vi "Initialize.vi"(8 "error in (no error)":errorcluster, 9 "Type":T1) -> (0 "error out":errorcluster, 1 "Stop Event":refnum<user-event>, 3 "UI_ProgressBar out":refnum<class "UI_ProgressDlg.lvclass">)   [LabVIEW 2014, in "UI_ProgressDlg.lvlib" / "UI_ProgressDlg.lvclass"]
uses:
  UI_ProgressDlg.lvclass
  _Control/DEF-Type.ctl
  _Control/DEF-Data.ctl
  UI_ProgressDlg.lvclass/UI_ProgressDlg.ctl
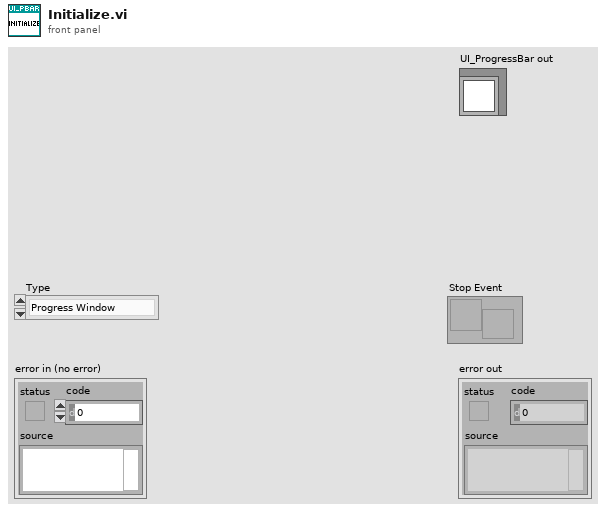
[diagram p1: front panel]
types:
  T1 = typedef "UI_ProgressDlg.lvlib/UI_ProgressDlg.lvclass/DEF-Type.ctl" = enum16{"Progress Window", "Buzy Window", "Timer Window"}
  T2 = typedef "UI_ProgressDlg.lvlib/UI_ProgressDlg.lvclass/DEF-Data.ctl" = cluster{"stopped?":bool}
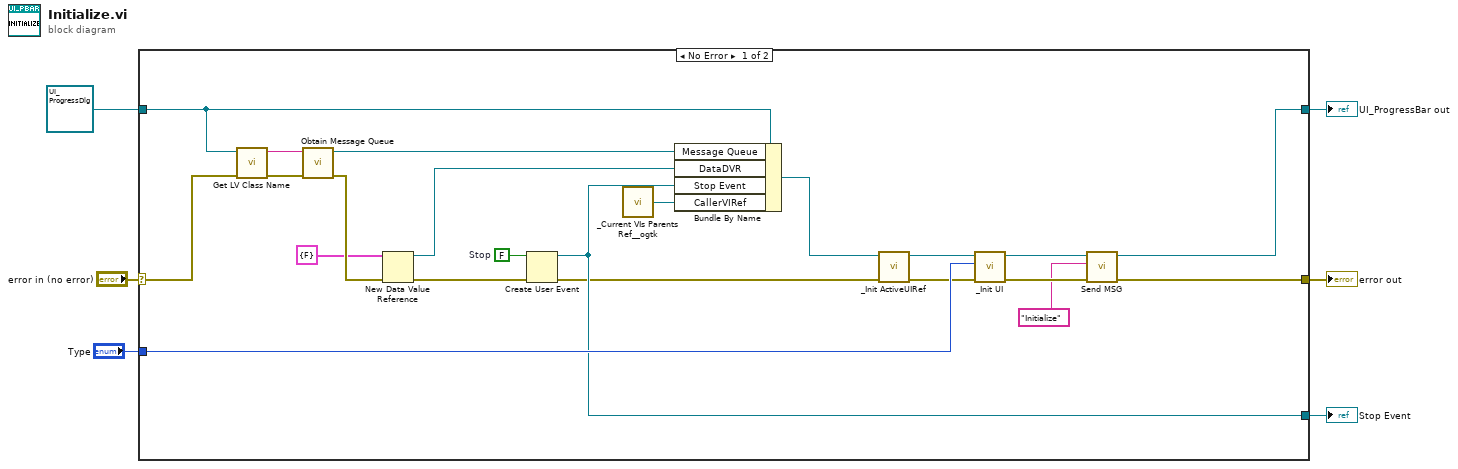
[diagram p0: block diagram]
diagram:
  n1 = case shown="No Error" "error in (no error)" {
    selector: "error in (no error)" -> [w28 w30]
    tunnel: [w17 w30] -> w5
    tunnel: [w19 w29] -> w3
    tunnel: refnum<class "UI_ProgressDlg.lvclass"> refnum ("UI_ProgressBar in") -> [w27 w29]
    tunnel: "Type" -> [w22 _]
    tunnel: [w13 _] -> w1
    frame No Error {
      w15 = FALSE  # Stop
      n2 = call <vilib>:"Get LV Class Name.vi"("error in (no error)"=w28, "object"=w27) -> ("error out"=w25:errorcluster, "class name"=w26:string)  [unwired: 8 in]
      n3 = call "Obtain Message Queue.vi"("error in (no error)"=w25, "name (unnamed)"=w26) -> ("error out"=w24:errorcluster, "Message Queue"=w23:refnum<queue>)  [unwired: 8 in]
      n4 = New Data Value Reference(data value=T2 {"stopped?"=FALSE} ("data"), error in=w24) -> (data value reference=w20:refnum<data-value>, error out=w14:errorcluster)
      n5 = Create User Event(user event datatype=w15, error in=w14) -> (user event=w13:refnum<user-event>, error out=w8:errorcluster)
      n6 = call "_Current VIs Parents Ref__ogtk.vi"() -> ("Calling VI's Reference"=w11:refnum<vi>)  [unwired: 2 in]
      n7 = Bundle By Name(cluster=w27, "Message Queue"=w23, "DataDVR"=w20, "Stop Event"=w13, "CallerVIRef"=w11) -> (w10:refnum<class "UI_ProgressDlg.lvclass">)
      n8 = call "_Init ActiveUIRef.vi"("error in (no error)"=w8, "UI_ProgressDlg in"=w10) -> ("error out"=w7:errorcluster, "UI_ProgressDlg out"=w9:refnum<class "UI_ProgressDlg.lvclass">)  [unwired: 8 in]
      n9 = call "_Init UI.vi"("error in (no error)"=w7, "Type"=w22, "UI_ProgressDlg in"=w9) -> ("error out"=w18:errorcluster, "UI_ProgressDlg out"=w12:refnum<class "UI_ProgressDlg.lvclass">)  [unwired: 7 in]
      n10 = call "Send MSG.vi"("error in (no error)"=w18, "msg"="Initialize", "UI_ProgressBar in"=w12) -> ("error out"=w17:errorcluster, "UI_ProgressBar out"=w19:refnum<class "UI_ProgressDlg.lvclass">)  [unwired: 7 in]
    }
    frame Error {
    }
  }
  "error out" <- w5
  "UI_ProgressBar out" <- w3
  "Stop Event" <- w1
